vi "(SubVI) Calculate PSD and Take Average_YCC.vi"(0 "Data":dbl[](array[numeric]), 2 "#samples per avg":dbl, 3 "Data rate (Hz)":dbl, 5 "T=NI made PSD\nF=YCC made PSD":bool) -> (6 "Avg. PSD":dbl[](array[numeric]), 8 "Frequency (Hz)\n0,df, 2df,...(n/2-1)Fs":dbl[](array[numeric]))   [LabVIEW 2014]
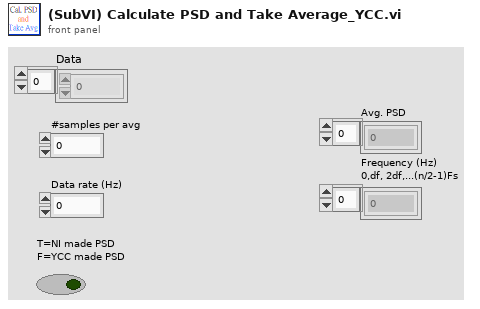
[diagram p1: front panel]
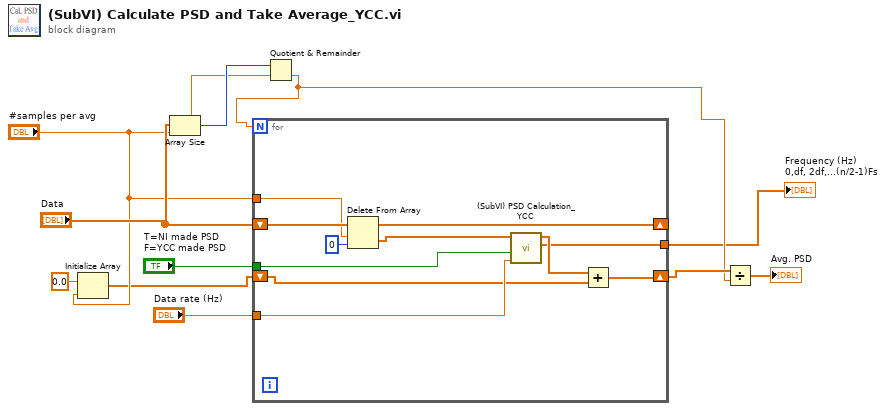
[diagram p0: block diagram]
diagram:
  n1 = Initialize Array(0.0 ("element"), "#samples per avg") -> (w5:dbl[])
  n2 = Array Size(array="Data") -> (size(s)=w9:i32)
  n3 = Quotient & Remainder(x=w9, y="#samples per avg") -> (floor(x/y)=w3:dbl)  [unwired: 1 out]
  n4 = for {
    N: w3 -> [_]
    tunnel: "Data rate (Hz)" -> [w21]
    tunnel: "#samples per avg" -> [w20]
    shift-right: [w18] -> _
    shift-left: "Data" -> [w22]
    tunnel: "T=NI made PSD\nF=YCC made PSD" -> [w16]
    shift-right: [w14] -> w4
    shift-left: w5 -> [w13]
    tunnel: [w12] -> w1
    n5 = Delete From Array(array=w22, length=w20, index=0) -> (deleted portion=w17:dbl[], array with subset deleted=w18:dbl[])
    n6 = call "(SubVI) PSD Calculation_YCC.vi"("sampling frequency (Hz)"=w21, "T=NI made PSD\nF=YCC made PSD"=w16, "QPD data"=w17) -> ("Frequency (Hz)\n0,df, 2df,...(n/2-1)Fs"=w12:dbl[], "Power Spectrum (V^2 rms) (V^2/Hz)"=w15:dbl[])  [unwired: 3 in]
    n7 = Add(x=w15, y=w13) -> (x+y=w14:dbl[])
  }
  "Frequency (Hz)\n0,df, 2df,...(n/2-1)Fs" <- w1
  n8 = Divide(x=w4, y=w3) -> (x/y=→"Avg. PSD":dbl[])
